vi "Z to dB, degrees.vi"   [LabVIEW 2020]
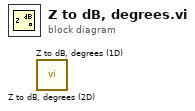
[diagram p0: block diagram]
diagram:
  n1 = call "Z to dB, degrees (2D).vi"() -> ()  [unwired: 6 in, 2 out]
  n2 = call "Z to dB, degrees (1D).vi"() -> ()  [unwired: 6 in, 2 out]
